vi "Begin.vi"(8 "error in":errorcluster) -> (0 "error out":errorcluster)   [LabVIEW 2019]
doc: "Called before other user functions, this VI is expected to open initial I/O refnums, load in file data, and do all program initialization. Notice that the <B>error out</B> terminal is simply used for data flow. Wiring it to other structures or subVIs ensures that this VI runs first."
uses:
  <vilib>/Rock Robotics/SystemInterfaces/DIO/FPGA_DIOPWMChannel.ctl
  <vilib>/Rock Robotics/WPI/SafetyOutput/WPI_SafetyOutputConfigMenu.ctl
  <vilib>/Rock Robotics/WPI/DriverStation/WPI_DriverStationRobotMode2.ctl
  <vilib>/Rock Robotics/WPI/Joystick/WPI_JoystickDeviceEnum.ctl
  <vilib>/Rock Robotics/SystemInterfaces/DIO/FPGA_DIOChannel.ctl
  <vilib>/Rock Robotics/SystemInterfaces/i2clib/i2c_bus.ctl
  <vilib>/Rock Robotics/WPI/RobotDrive/WPI_RobotDriveOpen2MotorWithTalon.vi
  Robot Global Data.vi
  <vilib>/Rock Robotics/Network Tables/NT Write String Array.vi
  <vilib>/Rock Robotics/WPI/Ultrasonic/WPI_SonarSRF04DigitalOpen.vi
  <vilib>/Rock Robotics/WPI/Ultrasonic/WPI_SonarSRF04DigitalRefNum Registry Set.vi
  <vilib>/Rock Robotics/WPI/MotorControl/WPI_MotorControlOpen VictorSP.vi
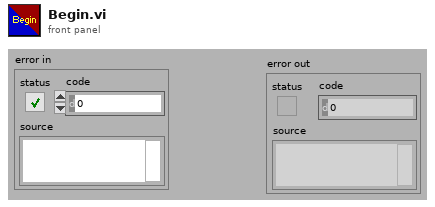
[diagram p1: front panel]
types:
  T1 = typedef "FPGA_DIOChannel.ctl" = enum8{"DIO 0", "DIO 1", "DIO 2", "DIO 3", "DIO 4", "DIO 5", "DIO 6", "DIO 7", "DIO 8", "DIO 9", "DIO MXP 0", "DIO MXP 1", "DIO MXP 2", "DIO MXP 3", "DIO MXP 4", "DIO MXP 5", "DIO MXP 6", "DIO MXP 7", "DIO MXP 8", "DIO MXP 9", "DIO MXP 10", "DIO MXP 11", "DIO MXP 12", "DIO MXP 13", "DIO MXP 14", "DIO MXP 15", "SPI Port CS1", "SPI Port CS2", "SPI Port CS3", "SPI Port MISO", "SPI Port MOSI", "Invalid"}
  T2 = typedef "FPGA_DIOPWMChannel.ctl" = enum8{"PWM 0", "PWM 1", "PWM 2", "PWM 3", "PWM 4", "PWM 5", "PWM 6", "PWM 7", "PWM 8", "PWM 9", "PWM MXP 0", "PWM MXP 1", "PWM MXP 2", "PWM MXP 3", "PWM MXP 4", "PWM MXP 5", "PWM MXP 6", "PWM MXP 7", "PWM MXP 8", "PWM MXP 9", "Invalid"}
  T3 = typedef "i2c_bus.ctl" = enum16{"I2C On-Board", "I2C MXP", "Invalid"}
  T4 = typedef "WPI_JoystickDeviceEnum.ctl" = enum16{"USB 0", "USB 1", "USB 2", "USB 3", "USB 4", "USB 5"}
  T5 = typedef "WPI_DriverStationRobotMode2.ctl" = enum16{"Autonomous Disabled", "Autonomous Enabled", "Teleop Disabled", "Teleop Enabled", "Disconnected", "Finish", "Test Disabled", "Test Enabled", "Emergency Stopped"}
  T6 = typedef "WPI_SafetyOutputConfigMenu.ctl" = enum16{"Enable", "Disable"}
  T7 = typedef "WPI_JoystickDevRef.ctl" = cluster{"Device":T4}
  T8 = typedef "WPI_RobotDriveDevRef.ctl" = cluster{"DevStatus":errorcluster, "Motors[]":T9[], "Square Inputs":bool, "Max Output":dbl}
  T9 = typedef "WPI_MotorControlDeviceRef.ctl" = cluster{"DeviceStatus":errorcluster, "Type":T10, "PWM":cluster{"PWM Channel":T2, "DeadBand":T11}, "CAN":cluster{"Device Number":u8, "SetOutput VI Ref":variant, "GetOutput VI Ref":variant, "Enable VI Ref":variant, "Disable VI Ref":variant, "Data":variant}, "Invert":bool, "DIO PWM":cluster{"PWM \"Enable\" Channel":T2, "DIOChannel":T1, "PWM Rate":dbl}}
  T10 = typedef "WPI_MotorControlType.ctl" = enum16{"PWM", "CAN", "DIO PWM"}
  T11 = typedef "WPI_PWMDeadband.ctl" = cluster{"Name":string, "maxPositivePwm":i32, "minPositivePwm":i32, "centerPwm":i32, "maxNegativePwm":i32, "minNegativePwm":i32, "angularRange":u16}
  T12 = typedef "WPI_UltrasonicDeviceRef.ctl" = cluster{"DevStatus":errorcluster, "Ping Channel":T1, "Echo Channel":T1, "CntIndex":T13}
  T13 = typedef "FPGA_CounterCtrSystemIndex.ctl" = enum8{"Ctr 0", "Ctr 1", "Ctr 2", "Ctr 3", "Ctr 4", "Ctr 5", "Ctr 6", "Ctr 7", "Invalid"}
  T14 = typedef "WPI_I2CDevRef.ctl" = cluster{"DevStatus":errorcluster, "Device Address":u8, "Handle":i32, "I2C Bus":T3}
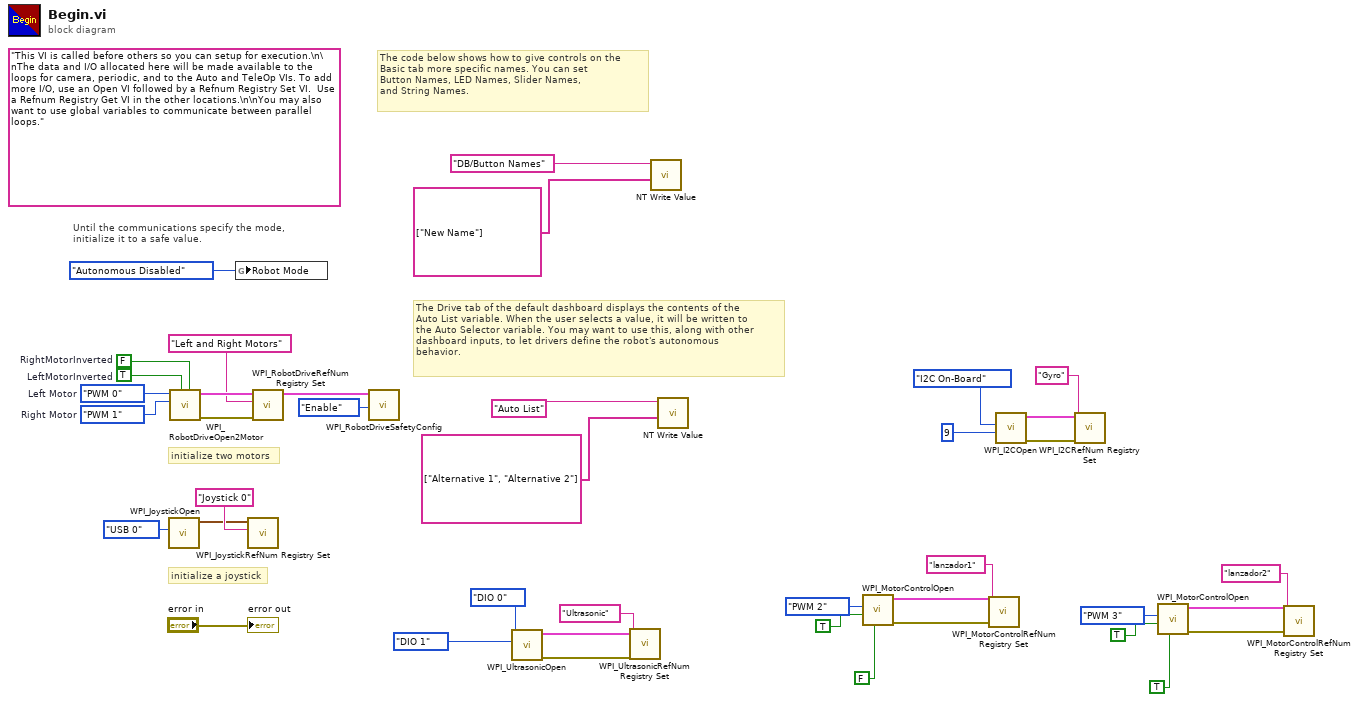
[diagram p0: block diagram]
diagram:
  (unwired) "This VI is called before others so you can setup for execution.\n\nThe data and I/O allocated here will be made available to the loops for camera, periodic, and to the Auto and TeleOp VIs. To add more I/O, use an Open VI followed by a Refnum Registry Set VI.  Use a Refnum Registry Get VI in the other locations.\n\nYou may also want to use global variables to communicate between parallel loops."
  w34 = FPGA_DIOPWMChannel."PWM 1"  # Right Motor
  w35 = FPGA_DIOPWMChannel."PWM 0"  # Left Motor
  w39 = TRUE  # LeftMotorInverted
  w40 = FALSE  # RightMotorInverted
  # "The Drive tab of the default dashboard displays the contents of the\nAuto List variable. When the user selects a value, it will be written to\nthe Auto Selector variable. You may want to use this, along with other\ndashboard inputs, to let drivers define the robot's autonomous\nbehavior."
  # "The code below shows how to give controls on the\nBasic tab more specific names. You can set\nButton Names, LED Names, Slider Names,\nand String Names."
  # "initialize a joystick"
  # "Until the communications specify the mode,\ninitialize it to a safe value."
  # "initialize two motors"
  n1 = call <vilib>:"WPI_JoystickOpen.vi"("JoystickDevice"=WPI_JoystickDeviceEnum."USB 0") -> ("JoystickDevRef"=w29:T7)  [unwired: 10 in]
  n2 = call-poly <vilib>:"WPI_RobotDriveOpen2Motor.vi"("Right Motor Inverted"=w40, "Left Motor Inverted"=w39, "Right Motor"=w34, "Left Motor"=w35) -> ("error out"=w36:errorcluster, "RobotDriveDevRef"=w38:T8)  [unwired: 1 in, 5 out]
  n3 = global write "Robot Global Data.vi" "Robot Mode"(WPI_DriverStationRobotMode2."Autonomous Disabled" ("Robot Mode")) -> ()
  n4 = call <vilib>:"WPI_JoystickRefNum Registry Set.vi"("refnum name"="Joystick 0", "JoystickDevRef"=w29) -> ()  [unwired: 8 in, 2 out]
  n5 = call <vilib>:"WPI_RobotDriveRefNum Registry Set.vi"("error in (no error)"=w36, "refnum name"="Left and Right Motors", "RobotDriveDevRef"=w38) -> ("RobotDriveDevRef"=w33:T8)  [unwired: 1 in, 7 out]
  n6 = call <vilib>:"WPI_RobotDriveSafetyConfig.vi"("mode"=WPI_SafetyOutputConfigMenu."Enable", "RobotDriveDevRef"=w33) -> ()  [unwired: 8 in, 2 out]
  n7 = call-poly <vilib>:"WPI_UltrasonicOpen.vi"("Echo DIO Channel"=FPGA_DIOChannel."DIO 1", "Ping DIO Channel"=FPGA_DIOChannel."DIO 0") -> ("error out"=w21:errorcluster, "SonarSRF04DevRef"=w22:T12)  [unwired: 8 in]
  n8 = call-poly <vilib>:"WPI_UltrasonicRefNum Registry Set.vi"("error in (no error)"=w21, "refnum name"="Ultrasonic", "SonarSRF04DevRef"=w22) -> ()  [unwired: 7 in, 2 out]
  n9 = call-poly <vilib>:"NT Write Value.vi"("String Array"=string[] ["New Name"], "Name"="DB/Button Names") -> ()  [unwired: 9 in, 1 out]
  n10 = call-poly <vilib>:"NT Write Value.vi"("String Array"=string[] ["Alternative 1", "Alternative 2"], "Name"="Auto List") -> ()  [unwired: 9 in, 1 out]
  n11 = call-poly <vilib>:"WPI_MotorControlOpen.vi"("Invert"=FALSE, "Eliminate Deadband"=TRUE, "PWM Channel"=FPGA_DIOPWMChannel."PWM 2") -> ("error out"=w9:errorcluster, "MotorControlDeviceRef"=w10:T9)  [unwired: 7 in]
  n12 = call <vilib>:"WPI_MotorControlRefNum Registry Set.vi"("error in (no error)"=w9, "refnum name"="lanzador1", "MotorControlDevRef"=w10) -> ()  [unwired: 7 in, 2 out]
  n13 = call <vilib>:"WPI_I2COpen.vi"("Device Address"=u8 9, "I2C Bus"=i2c_bus."I2C On-Board") -> ("error out"=w15:errorcluster, "I2CDevRef"=w16:T14)  [unwired: 8 in]
  n14 = call <vilib>:"WPI_I2CRefNum Registry Set.vi"("error in (no error)"=w15, "refnum name"="Gyro", "I2CDevRef"=w16) -> ()  [unwired: 7 in, 2 out]
  n15 = call-poly <vilib>:"WPI_MotorControlOpen.vi"("Invert"=TRUE, "Eliminate Deadband"=TRUE, "PWM Channel"=FPGA_DIOPWMChannel."PWM 3") -> ("error out"=w3:errorcluster, "MotorControlDeviceRef"=w4:T9)  [unwired: 7 in]
  n16 = call <vilib>:"WPI_MotorControlRefNum Registry Set.vi"("error in (no error)"=w3, "refnum name"="lanzador2", "MotorControlDevRef"=w4) -> ()  [unwired: 7 in, 2 out]
  "error out" <- "error in"
